vi "Add new Exchange Map.vi"() -> (8 "Long":string, 9 "Lat":string, 10 "Name of University":string, 11 "table id":string)   [LabVIEW 2010]
uses:
  <vilib>/Utility/file.llb/Read From Spreadsheet File (string).vi
panel:
  out "name of logo":string
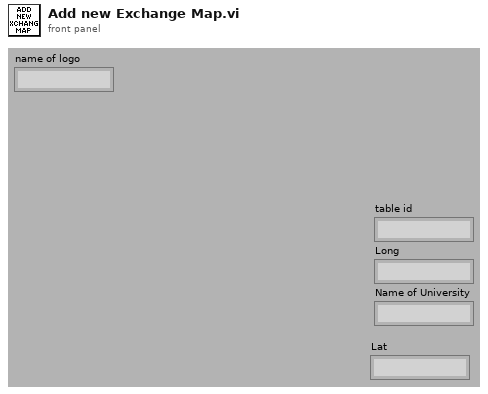
[diagram p1: front panel]
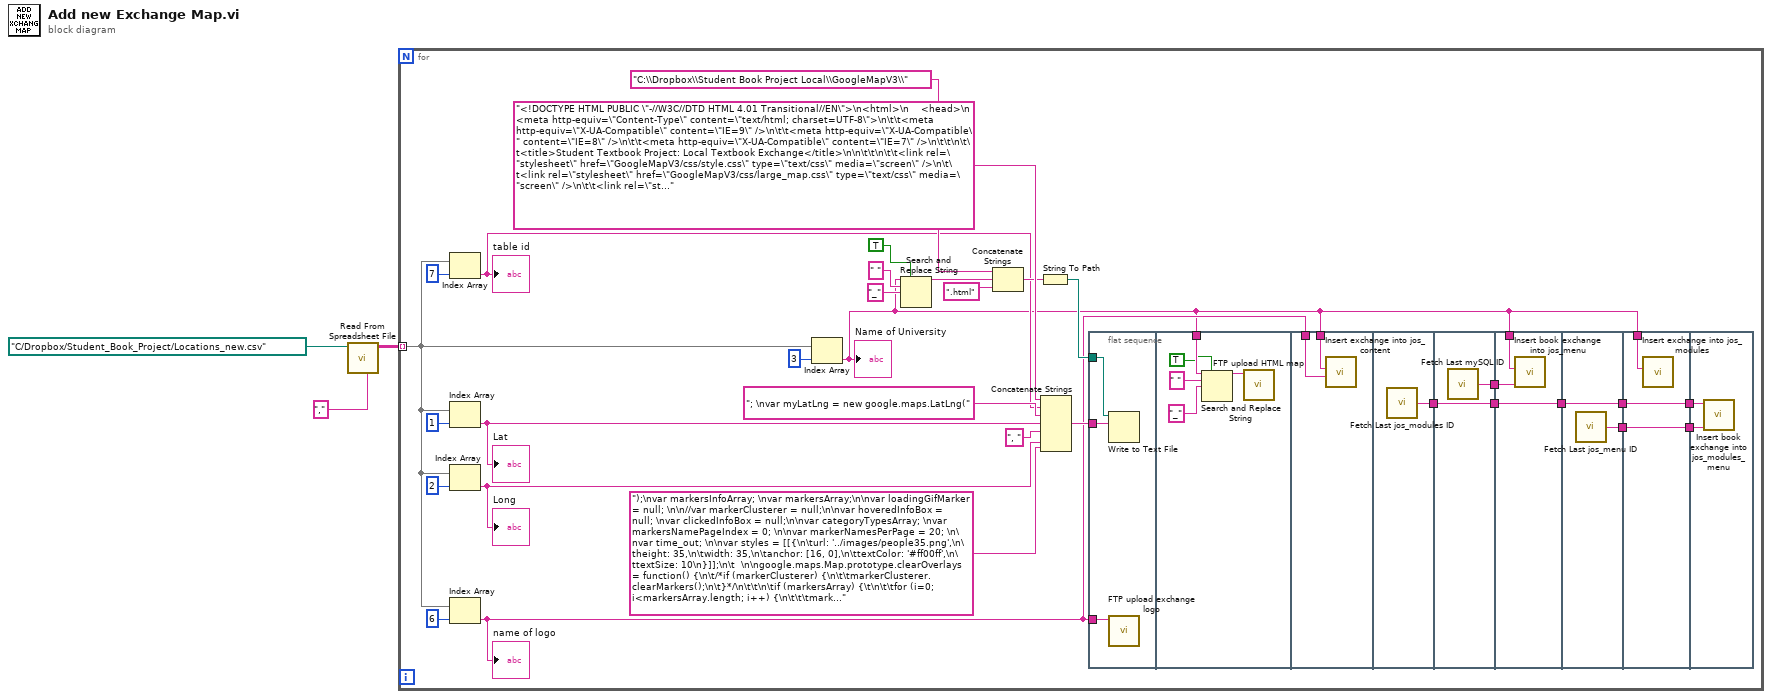
[diagram p0: block diagram]
diagram:
  n1 = call-poly <vilib>:"Read From Spreadsheet File.vi"("delimiter (\\t)"="," ("delimiter (\\t)"), "file path (dialog if empty)"=path "C:/Dropbox/Student_Book_Project/Locations_new.csv") -> ("all rows"=w1:string[][])  [unwired: 5 in, 4 out]
  n2 = for {
    tunnel: w1 -> [w6] mode=indexing
    n3 = Index Array(array=w6, index=7) -> (element=w5:string)
    "table id" <- w5
    n4 = Index Array(array=w6, index=1) -> (element=w13:string)
    "Lat" <- w13
    n5 = Index Array(array=w6, index=2) -> (element=w11:string)
    "Long" <- w11
    n6 = Index Array(array=w6, index=6) -> (element=w7:string)
    "name of logo" <- w7
    n7 = Index Array(array=w6, index=3) -> (element=w4:string)
    "Name of University" <- w4
    n8 = Search and Replace String(replace all?=TRUE ("replace all? (F)"), input string=w4, search string=" ", replace string="_" ("replace string (\"\")")) -> (result string=w15:string)  [unwired: 4 in, 3 out]
    n9 = Concatenate Strings("C:\\Dropbox\\Student Book Project Local\\GoogleMapV3\\", w15, ".html" ("string")) -> (w21:string)
    n10 = String To Path(string=w21) -> (path=w19:path)
    n11 = Concatenate Strings("<!DOCTYPE HTML PUBLIC \"-//W3C//DTD HTML 4.01 Transitional//EN\">\n<html>\n    <head>\n        <meta http-equiv=\"Content-Type\" content=\"text/html; charset=UTF-8\">\n\t\t<meta http-equiv=\"X-UA-Compatible\" content=\"IE=9\" />\n\t\t<meta http-equiv=\"X-UA-Compatible\" content=\"IE=8\" />\n\t\t<meta http-equiv=\"X-UA-Compatible\" content=\"IE=7\" />\n\t\t\n\t\t<title>Student Textbook Project: Local Textbook Exchange</title>\n\n\t\t\n\t\t<link rel=\"stylesheet\" href=\"GoogleMapV3/css/style.css\" type=\"text/css\" media=\"screen\" />\n\t\t<link rel=\"stylesheet\" href=\"GoogleMapV3/css/large_map.css\" type=\"text/css\" media=\"screen\" />\n\t\t<link rel=\"stylesheet\" href=\"GoogleMapV3/css/jquery.customSelect.css\" type=\"text/css\" media=\"screen\" />\n\t\t<link href='http://fonts.googleapis.com/css?family=Happy+Monkey' rel='stylesheet' type='text/css'>\n\t\t<link href='http://fonts.googleapis.com/css?family=Lobster' rel='stylesheet' type='text/css'>\n\t\t<script type=\"text/javascript\" src=\"https://ajax.googleapis.com/ajax/libs/jquery/1.7.1/jquery.min.js\"></script>\n\t\t<!--<script type='text/javascript' src='GoogleMapV3/js/easing.js'></script>-->\n\t\t<script type=\"text/javascript\" src=\"http://maps.google.com/maps/api/js?sensor=false\"></script>\n\t\t<script type=\"text/javascript\" src=\"http://www.google.com/jsapi\"></script>\t\n\n        <script type=\"text/javascript\">\n\t\tvar map;\nvar tableid = ", w5, "; \nvar myLatLng = new google.maps.LatLng(" ("string"), w13, ", " ("string"), w11, ");\nvar markersInfoArray; \nvar markersArray;\n\nvar loadingGifMarker = null; \n\n//var markerClusterer = null;\n\nvar hoveredInfoBox = null; \nvar clickedInfoBox = null;\n\nvar categoryTypesArray; \nvar markersNamePageIndex = 0; \n\nvar markerNamesPerPage = 20; \n\nvar time_out; \n\nvar styles = [[{\n\turl: '../images/people35.png',\n\theight: 35,\n\twidth: 35,\n\tanchor: [16, 0],\n\ttextColor: '#ff00ff',\n\ttextSize: 10\n}]];\n\t  \n\ngoogle.maps.Map.prototype.clearOverlays = function() {\n\t/*if (markerClusterer) {\n\t\tmarkerClusterer.clearMarkers();\n\t}*/\n\t\t\n\tif (markersArray) {\t\n\t\tfor (i=0; i<markersArray.length; i++) {\n\t\t\tmarkersArray[i].setMap(null);\n\t\t}\n\t}\n}\n\ngoogle.load('visualization', '1');\n\n\nfunction initialize()\n{\t\n\t$(\"#controlbtn\").click(function(e) {\n\t\te.preventDefault();\n\t\t\n\t\tvar slidepx=$(\"#srp_left_rail\").width();\n\t\t\n\t\tif ( !$(\"#large_map\").is(':animated') ) { \n\t\t\tif (Math.abs(parseInt($(\"#large_map\").css('marginLeft'), 10)) < slidepx) {\n\t\t\t\t$(this).removeClass('close').html('Hide your stuffs');\n\t\t\t\t\n\t\t\t\tmargin = \"-=\" + slidepx;\n\n\t\t\t} else {\n\t\t\t\t$(this).addClass('close').html('Show your stuffs');\n\t\t\t\t\n\t\t\t\tmargin = \"+=\" + slidepx;\n\n\t\t\t}\n\t\t\n\t\t\t$(\"#large_map\").animate({ \n\t\t\t\tmarginLeft: margin\n\t\t\t}, {\n\t\t\t\t\tduration: 'slow',\n\t\t\t\t\teasing: 'easeOutQuint'\n\t\t\t\t});\t\t\t\t\t\n\t\t} \n\t});\n\t\n\tvar myOptions = {\n\t\tzoom: 14,\n\t\tcenter: myLatLng,\n\t\tmapTypeId: google.maps.MapTypeId.ROADMAP\n\t};\n\tmap = new google.maps.Map(document.getElementById(\"map_canvas\"), myOptions);\n\t\n\tvar query = \"SELECT 'Lat', 'Lng', 'Title', 'Category', 'Price', 'ID' FROM \" + tableid;\n\t\n\tvar queryText = encodeURIComponent(query);\n\tvar gvizQuery = new google.visualization.Query('http://www.google.com/fusiontables/gvizdata?tq=' + queryText);\n\t\n\tmarkersNamePageIndex = 0; \n\tgvizQuery.send(function(response) { \t\n\t\tvar numRows = response.getDataTable().getNumberOfRows();\n\t\t\n\t\t// create the list of lat/long coordinates\n\t\tmarkersInfoArray = [];\n\t\tvar coordinates = [];\n\t\tcategoryTypesArray = [];\n\t\t\n\t\tfor (i=0; i<numRows; i++) {\n\t\t\tvar lat = parseFloat(response.getDataTable().getValue(i, 0));\n\t\t\tvar lng = parseFloat(response.getDataTable().getValue(i, 1));\n\t\t\tvar title = response.getDataTable().getValue(i, 2);\n\t\t\tvar category = response.getDataTable().getValue(i, 3);\n\t\t\tvar price = response.getDataTable().getValue(i, 4);\n\t\t\tvar id = response.getDataTable().getValue(i, 5);\n\t\t\t\n\t\t\tcoordinates.push(new google.maps.LatLng(lat, lng));\n\t\t\n\t\t\tmarkersInfoArray[i] = {id:id, lat:lat, lng:lng, title:title, category:category, price:price};\n\t\t\t\n\t\t\tif (!categoryTypesArray.contains(category)) {\n\t\t\t\tcategoryTypesArray.push(category);\n\t\t\t}\n\t\t}\t\t\t\t\t\n\t\trefreshMarkersCategoryList();\n\t\t\n\t\tmap.clearOverlays();\n\t\tmarkersArray = [];\n\t\t\n\t\tfor (i=0; i<coordinates.length; i++) {\n\t\t\tvar latLng = coordinates[i];\n\t\t\tif (latLng == null) continue; \n\t\t\t\n\t\t\tvar markerInfo = markersInfoArray[i];\n\t\t\tcreateMarker(markerInfo, latLng);\n\t\t}\n\t\t\n\t\t/*var zoom = null; var size = null; var style = null; \n        markerClusterer = new MarkerClusterer(map, markersArray, {\n\t\t\tmaxZoom: zoom,\n\t\t\tgridSize: size,\n\t\t\tstyles: styles[style]\n        });*/\n\t\t\n\t\tvar bounds = new google.maps.LatLngBounds();\n\t\tfor (var i = 0; i < coordinates.length; i++) {\n\t\t\tbounds.extend(coordinates[i]);\n\t\t}\n\t\t\n\t\trefreshMarkersNameList();\n\t});\n}\n\nfunction createMarker(markerInfo, latlng) {\n\tvar id = markerInfo.id;\n\tvar category = markerInfo.category; \n\tvar lat = markerInfo.lat; \n\tvar lng = markerInfo.lng;\n\tvar latLng = new google.maps.LatLng(lat, lng);\n\t\n\tvar color = \"0000FF\"; \n\tif (category == \"History\")\n\t\tcolor = \"0000FF\";\n\telse if (category == \"Film Studies\")\n\t\tcolor = \"FF0000\";\n\telse if (category == \"Biology\")\n\t\tcolor = \"FF9900\"\n\telse if (category == \"Engineering\")\n\t\tcolor = \"E661AC\";\t\t\t\t\t\n\telse if (category == \"Education\")\n\t\tcolor = \"BF94E4\";\n\telse if (category == \"Music\")\n\t\tcolor = \"8E67FD\";\n\telse if (category == \"Chemistry\")\n\t\tcolor = \"804040\";\n\telse if (category == \"Economics\")\n\t\tcolor = \"FF8300\";\n\telse if (category == \"Political Science\")\n\t\tcolor = \"000000\";\n\telse if (category == \"Medical\")\n\t\tcolor = \"00FF00\";\n\telse if (category == \"Mathematics\")\n\t\tcolor = \"06DCFB\";\t\n\telse if (category == \"Psychology\")\n\t\tcolor = \"FF68DD\"; \n\telse if (category == \"Uncategorized\")\n\t\tcolor = \"1FCB4A\";\n\telse if (category == \"Physics\")\n\t\tcolor = \"800080\"; \n\telse if (category == \"Language\")\n\t\tcolor = \"804040\"; \n\telse if (category == \"Hospitality Management\")\n\t\tcolor = \"988727\"; \n\telse if (category == \"Nursing\")\n\t\tcolor = \"808080\"; \n\telse if (category == \"Business\")\n\t\tcolor = \"0080FF\"; \n\telse if (category == \"Art\")\n\t\tcolor = \"FF8080\"; \n\t\n\tvar markerString = markerInfo.price.toString();\n\t\n\tvar marker = new google.maps.Marker({\n\t\tposition: latlng,\n\t\tdraggable: false,\n\t\tmap: map,\n\t\ticon: new google.maps.MarkerImage(\"http://chart.googleapis.com/chart?chst=d_bubble_text_small&chld=bb|\"+markerString+\"|\"+color+\"|FFFFFF\", null, null, new google.maps.Point(15, 42)),\n\t\tshadow: new google.maps.MarkerImage(\"http://chart.googleapis.com/chart?chst=d_bubble_text_small_shadow&chld=bb|\"+markerString, null, null, new google.maps.Point(15, 45))\n\t});\n\tmarker.set(\"id\", id);\n\t\n\tmarkersArray.push(marker);\t\t\t\t\n\t\n\t// when hovering the bookstore ...\t\n\tgoogle.maps.event.addListener(marker, \"mouseover\", function(e) {\n\t\tvar id = marker.get(\"id\");\n\t\tvar query = \"SELECT 'Date', 'Time', 'Lat', 'Lng', 'Title', 'Category', 'Author', 'ISBN', 'Price', 'Class Identifier', 'Condition', 'Contact Info', 'Meta', 'Extra Information', 'Username', 'UserID', 'Name', 'Address', 'City', 'State', 'Zip Code', 'Country', 'timestamp', 'ID' FROM \" + tableid + \" WHERE ID='\" + id + \"'\";\n\t\t\n\t\tvar queryText = encodeURIComponent(query);\n\t\tvar gvizQuery = new google.visualization.Query('http://www.google.com/fusiontables/gvizdata?tq=' + queryText);\n\t\t\n\t\tgvizQuery.send(function(response) { \t\n\t\t\tvar numRows = response.getDataTable().getNumberOfRows();\n\t\t\t\n\t\t\tfor (i=0; i<numRows; i++) {\n\t\t\t\tvar date = response.getDataTable().getValue(i, 0);\n\t\t\t\tvar time = response.getDataTable().getValue(i, 1);\n\t\t\t\tvar lat = parseFloat(response.getDataTable().getValue(i, 2));\n\t\t\t\tvar lng = parseFloat(response.getDataTable().getValue(i, 3));\n\t\t\t\tvar title = response.getDataTable().getValue(i, 4);\n\t\t\t\tvar category = response.getDataTable().getValue(i, 5);\n\t\t\t\tvar author = response.getDataTable().getValue(i, 6);\n\t\t\t\tvar isbn = response.getDataTable().getValue(i, 7);\n\t\t\t\tvar price = response.getDataTable().getValue(i, 8);\n\t\t\t\tvar class_identifier = response.getDataTable().getValue(i, 9);\n\t\t\t\tvar condition = response.getDataTable().getValue(i, 10);\n\t\t\t\tvar contact_info = response.getDataTable().getValue(i, 11);\n\t\t\t\tvar meta = response.getDataTable().getValue(i, 12);\n\t\t\t\tvar extra_information = response.getDataTable().getValue(i, 13);\n\t\t\t\tvar username = response.getDataTable().getValue(i, 14);\n\t\t\t\tvar userid = response.getDataTable().getValue(i, 15);\n\t\t\t\tvar name = response.getDataTable().getValue(i, 16);\n\t\t\t\tvar address = response.getDataTable().getValue(i, 17);\n\t\t\t\tvar city = response.getDataTable().getValue(i, 18);\n\t\t\t\tvar state = response.getDataTable().getValue(i, 19);\n\t\t\t\tvar zipcode = response.getDataTable().getValue(i, 20);\n\t\t\t\tvar country = response.getDataTable().getValue(i, 21);\n\t\t\t\tvar timestamp = response.getDataTable().getValue(i, 22);\n\t\t\t\tvar id = response.getDataTable().getValue(i, 23);\n\t\t\t\t\n\t\t\t\tvar hoveredBoxText = document.createElement(\"div\");\n\t\t\t\thoveredBoxText.style.cssText = \"border: 1px solid black; margin-top: 8px; background:#333; color:#FFF; font-family: 'Happy Monkey', cursive; font-size:12px; padding: 5px; border-radius:8px; -moz-border-radius:8px; -webkit-border-radius:8px; behavior: url(ie-css3.htc);\";\n\t\t\t\thoveredBoxText.innerHTML = '<div style=\"height:400px; overflow:auto;\"><p style=\"font-size:16px; font-weight:bold; color:#3990BD; margin-top:0px; margin-bottom:-10px;\">' + title + '</p>' + \n\t\t\t\t\t\t\t\"<br /><br /><strong>Category</strong>:  \" + category + \n\t\t\t\t\t\t\t\"<br /><strong>Author</strong>:  \" + author + \n\t\t\t\t\t\t\t\"<br /><strong>ISBN</strong>:  \" + isbn + \n\t\t\t\t\t\t\t\"<br /><strong>Price</strong>:  \" + price + \n\t\t\t\t\t\t\t\"<br /><strong>Class Identifier</strong>:  \" + class_identifier + \n\t\t\t\t\t\t\t\"<br /><strong>Condition</strong>:  \" + condition + \n\t\t\t\t\t\t\t\"<br /><strong>Contact Info</strong>:  \" + contact_info + \n\t\t\t\t\t\t\t\"<br />  \" + extra_information + '</div>';\n\t\t\t\t\n\t\t\t\tvar hoveredInfoBoxOptions = {\n\t\t\t\t\tcontent: hoveredBoxText\n\t\t\t\t\t,disableAutoPan: false\n\t\t\t\t\t,maxWidth: 0\n\t\t\t\t\t,pixelOffset: new google.maps.Size(-133, 0)\n\t\t\t\t\t,zIndex: 100000\n\t\t\t\t\t,boxStyle: { \n\t\t\t\t\t\tbackground: \"url('GoogleMapV3/images/tipbox.gif') no-repeat\"\n\t\t\t\t\t\t,opacity: 0.94\n\t\t\t\t\t\t,width: \"350px\"\n\t\t\t\t\t\t,height: \"400px\"\t\t\t\t\t\t\t\n\t\t\t\t\t}\n\t\t\t\t\t,closeBoxMargin: \"15px 7px 7px 7px\"\n\t\t\t\t\t,closeBoxURL: \"http://www.google.com/intl/en_us/mapfiles/close.gif\"\n\t\t\t\t\t,infoBoxClearance: new google.maps.Size(1, 1)\n\t\t\t\t\t,isHidden: false\n\t\t\t\t\t,pane: \"floatPane\"\n\t\t\t\t\t,enableEventPropagation: false\n\t\t\t\t\t,disableAutoPan: true\n\t\t\t\t};\n\t\t\t\t\n\t\t\t\tif (hoveredInfoBox != null)\n\t\t\t\t\thoveredInfoBox.close(); \n\t\t\t\t\t\t\n\t\t\t\tif (hoveredInfoBox == null)\n\t\t\t\t\thoveredInfoBox = new InfoBox(hoveredInfoBoxOptions);\n\t\t\t\telse {\n\t\t\t\t\thoveredInfoBox.setContent(hoveredBoxText);\t\t\t\t\t\t\n\t\t\t\t\thoveredInfoBox.setZIndex(100000);\n\t\t\t\t}\n\t\t\t\t\t\n\t\t\t\thoveredInfoBox.setContent(hoveredBoxText);\t\t\t\t\t\t\n\t\t\t\thoveredInfoBox.setZIndex(100000);\n\t\t\t\thoveredInfoBox.open(map, marker);\n\t\t\t}\n\t\t});\n\t});\n\t\n\tgoogle.maps.event.addListener(marker, \"mouseout\", function(e) {\t\t\n\t\thoveredInfoBox.close();\n\t});\n\t\n\t// when clicking the bookstore ...\t\n\tgoogle.maps.event.addListener(marker, \"click\", function(e) {\n\t\tvar id = marker.get(\"id\");\n\t\tvar query = \"SELECT 'Date', 'Time', 'Lat', 'Lng', 'Title', 'Category', 'Author', 'ISBN', 'Price', 'Class Identifier', 'Condition', 'Contact Info', 'Meta', 'Extra Information', 'Username', 'UserID', 'Name', 'Address', 'City', 'State', 'Zip Code', 'Country', 'timestamp', 'ID' FROM \" + tableid + \" WHERE ID='\" + id + \"'\";\n\t\t\n\t\tvar queryText = encodeURIComponent(query);\n\t\tvar gvizQuery = new google.visualization.Query('http://www.google.com/fusiontables/gvizdata?tq=' + queryText);\n\t\t\n\t\tgvizQuery.send(function(response) { \t\n\t\t\tvar numRows = response.getDataTable().getNumberOfRows();\n\t\t\t\n\t\t\tfor (i=0; i<numRows; i++) {\n\t\t\t\tvar date = response.getDataTable().getValue(i, 0);\n\t\t\t\tvar time = response.getDataTable().getValue(i, 1);\n\t\t\t\tvar lat = parseFloat(response.getDataTable().getValue(i, 2));\n\t\t\t\tvar lng = parseFloat(response.getDataTable().getValue(i, 3));\n\t\t\t\tvar title = response.getDataTable().getValue(i, 4);\n\t\t\t\tvar category = response.getDataTable().getValue(i, 5);\n\t\t\t\tvar author = response.getDataTable().getValue(i, 6);\n\t\t\t\tvar isbn = response.getDataTable().getValue(i, 7);\n\t\t\t\tvar price = response.getDataTable().getValue(i, 8);\n\t\t\t\tvar class_identifier = response.getDataTable().getValue(i, 9);\n\t\t\t\tvar condition = response.getDataTable().getValue(i, 10);\n\t\t\t\tvar contact_info = response.getDataTable().getValue(i, 11);\n\t\t\t\tvar meta = response.getDataTable().getValue(i, 12);\n\t\t\t\tvar extra_information = response.getDataTable().getValue(i, 13);\n\t\t\t\tvar username = response.getDataTable().getValue(i, 14);\n\t\t\t\tvar userid = response.getDataTable().getValue(i, 15);\n\t\t\t\tvar name = response.getDataTable().getValue(i, 16);\n\t\t\t\tvar address = response.getDataTable().getValue(i, 17);\n\t\t\t\tvar city = response.getDataTable().getValue(i, 18);\n\t\t\t\tvar state = response.getDataTable().getValue(i, 19);\n\t\t\t\tvar zipcode = response.getDataTable().getValue(i, 20);\n\t\t\t\tvar country = response.getDataTable().getValue(i, 21);\n\t\t\t\tvar timestamp = response.getDataTable().getValue(i, 22);\n\t\t\t\tvar id = response.getDataTable().getValue(i, 23);\n\t\t\t\t\n\t\t\t\t// clicked info bubble ...\n\t\t\t\tvar clickedBoxText = document.createElement(\"div\");\n\t\t\t\tclickedBoxText.style.cssText = \"border: 1px solid black; margin-top: 8px; background:#333; color:#FFF; font-family: 'Happy Monkey', cursive; font-size:12px; padding: 5px; border-radius:8px; -webkit-border-radius:8px; -moz-border-radius:8px;\";\n\t\t\t\tclickedBoxText.innerHTML = '<div style=\"height:400px; overflow:auto;\"><p style=\"font-size:16px; font-weight:bold; color:#3990BD; margin-top:0px; margin-bottom:-10px;\">' + title + '</p>' + \n\t\t\t\t\t\t\t\"<br /><br /><strong>Category</strong>:  \" + category + \n\t\t\t\t\t\t\t\"<br /><strong>Author</strong>:  \" + author + \n\t\t\t\t\t\t\t\"<br /><strong>ISBN</strong>:  \" + isbn + \n\t\t\t\t\t\t\t\"<br /><strong>Price</strong>:  \" + price + \n\t\t\t\t\t\t\t\"<br /><strong>Class Identifier</strong>:  \" + class_identifier + \n\t\t\t\t\t\t\t\"<br /><strong>Condition</strong>:  \" + condition + \n\t\t\t\t\t\t\t\"<br /><strong>Contact Info</strong>:  \" + contact_info + \n\t\t\t\t\t\t\t\"<br />  \" + extra_information + '</div>';\n\t\t\t\t\n\t\t\t\tvar clickedInfoBoxOptions = {\n\t\t\t\t\tcontent: clickedBoxText\n\t\t\t\t\t,disableAutoPan: false\n\t\t\t\t\t,maxWidth: 0\n\t\t\t\t\t,pixelOffset: new google.maps.Size(-133, 0)\n\t\t\t\t\t,zIndex: 100000\n\t\t\t\t\t,boxStyle: { \n\t\t\t\t\t\tbackground: \"url('GoogleMapV3/images/tipbox.gif') no-repeat\"\n\t\t\t\t\t\t,opacity: 0.94\n\t\t\t\t\t\t,width: \"400px\"\n\t\t\t\t\t\t,height: \"450px\"\t\t\t\t\t\t\t\n\t\t\t\t\t}\n\t\t\t\t\t,closeBoxMargin: \"15px 7px 7px 7px\"\n\t\t\t\t\t,closeBoxURL: \"http://www.google.com/intl/en_us/mapfiles/close.gif\"\n\t\t\t\t\t,infoBoxClearance: new google.maps.Size(1, 1)\n\t\t\t\t\t,isHidden: false\n\t\t\t\t\t,pane: \"floatPane\"\n\t\t\t\t\t,enableEventPropagation: false\n\t\t\t\t};\n\t\t\t\t\n\t\t\t\tif (clickedInfoBox == null)\n\t\t\t\t\tclickedInfoBox = new InfoBox(clickedInfoBoxOptions);\n\t\t\t\telse {\n\t\t\t\t\tclickedInfoBox.setContent(clickedBoxText);\t\t\t\t\t\t\n\t\t\t\t\tclickedInfoBox.setZIndex(100000);\n\t\t\t\t}\n\t\t\t\t\n\t\t\t\tif (hoveredInfoBox != null)\n\t\t\t\t\thoveredInfoBox.close(); \n\t\t\t\tif (clickedInfoBox != null)\n\t\t\t\t\tclickedInfoBox.close();\n\t\t\t\t\t\n\t\t\t\tclickedInfoBox.setContent(clickedBoxText);\t\t\t\t\t\t\n\t\t\t\tclickedInfoBox.setZIndex(100000);\n\t\t\t\t\n\t\t\t\tclickedInfoBox.open(map, marker);\n\t\t\t}\n\t\t});\n\t});\n}\n\nfunction refreshMarkersCategoryList() { \n\tcategoryTypesArray.sort(sortNumber);\n\t\n\tvar marker_categories_select = document.getElementById('marker_categories');\n\taddSelectOption(marker_categories_select, \"All\", 0, true);\n\t\n\tfor (i=0; i<categoryTypesArray.length; i++) {\n\t\tvar added_current_category = categoryTypesArray[i];\n\t\taddSelectOption(marker_categories_select, added_current_category, added_current_category, false);\n\t}\n} \n\nfunction refreshMarkersNameList() { \n\t\n\tvar marker_titles_add_html = \"\";\t\t\t\t\n\t\n\tvar markersNum = markersInfoArray.length; \n\tvar markerInfo; var markerName; var markerId; \n\tif (markersNum > markerNamesPerPage) {\n\t\tfor (i=0; i<markerNamesPerPage; i++) {\n\t\t\tif ( (i + markersNamePageIndex * markerNamesPerPage) >= markersNum )\n\t\t\t\tbreak;\n\t\t\t\t\n\t\t\tmarkerInfo = markersInfoArray[i + markersNamePageIndex * markerNamesPerPage];\n\t\t\tmarkerTitle = markerInfo.title; \n\t\t\tmarkerId = markerInfo.id;\n\t\t\t\n\t\t\tmarker_titles_add_html += '<li><a title=\"' + markerTitle + '\" href=\"javascript:void(0);\" onmouseover=\"openMarkerNameInfoWindowOnMap(' + markerId + ')\" onmouseout=\"closeMarkerNameInfoWindowOnMap(' + markerId + ')\" onclick=\"selectMarkerInfoOnMap(' + markerId + ')\">' + markerTitle + '</a></li>'\n\t\t}\n\t\t\n\t\tvar marker_names_prev_next_html = \"\";\n\t\tmarker_names_prev_next_html += '<a href=\"javascript:void(0);\" onclick=\"showPrevMarkerNames();\" style=\"margin-left:40px;\"><< Previous</a>'\n\t\tmarker_names_prev_next_html += '<a href=\"javascript:void(0);\" onclick=\"showNextMarkerNames();\" style=\"margin-left:60px;\">Next >></a>'\n\n\t\tdocument.getElementById('markers_prev_next_section').innerHTML = marker_names_prev_next_html; \n\t} else {\n\t\tfor (i=0; i<markersNum; i++) {\n\t\t\tmarkerInfo = markersInfoArray[i];\n\t\t\tmarkerTitle = markerInfo.title; \n\t\t\tmarkerId = markerInfo.id;\n\t\t\t\n\t\t\tmarker_titles_add_html += '<li><a title=\"' + markerName + '\" href=\"javascript:void(0);\" onmouseover=\"openMarkerNameInfoWindowOnMap(' + markerId + ')\" onmouseout=\"closeMarkerNameInfoWindowOnMap(' + markerId + ')\" onclick=\"selectMarkerInfoOnMap(' + markerId + ')\">' + markerTitle + '</a></li>'\n\t\t}\n\t\t\n\t\tdocument.getElementById('markers_prev_next_section').innerHTML = \"\"; \n\t}\n\tdocument.getElementById('markers_list').innerHTML = marker_titles_add_html; \n}\n\nfunction showPrevMarkerNames() { \n\tif (markersNamePageIndex == 0)\n\t\treturn;\n\t\t\n\tmarkersNamePageIndex--;\n\trefreshMarkersNameList();\n}\n\nfunction showNextMarkerNames() { \n\tvar markersNum = markersInfoArray.length; \n\tif ( ((markersNamePageIndex+1) * markerNamesPerPage) > markersNum ) \n\t\treturn; \n\t\t\n\tmarkersNamePageIndex++;\n\trefreshMarkersNameList();\n}\n\nfunction SearchBooks(search_text, search_category) {\n\tsearch_text = trim(search_text.toString());\n\t\n\tvar query = \"\"; \n\t\n\tif (search_category == 0)\n\t\tquery = \"SELECT 'Lat', 'Lng', 'Title', 'Category', 'Price', 'ID' FROM \" + tableid;\n\telse \n\t\tquery = \"SELECT 'Lat', 'Lng', 'Title', 'Category', 'Price', 'ID' FROM \" + tableid + \" WHERE Category='\" + search_category.toString() + \"'\";\n\t\t\n\tvar queryText = encodeURIComponent(query);\n\tvar gvizQuery = new google.visualization.Query('http://www.google.com/fusiontables/gvizdata?tq='  + queryText);\n\t\n\tmarkersNamePageIndex = 0; \n\t\n\t// Send query and draw table with data in response\n\tgvizQuery.send(function(response) {\n\t\tvar numRows = response.getDataTable().getNumberOfRows();\n\t\tvar numCols = response.getDataTable().getNumberOfColumns();\n\t\t\n\t\t// create the list of lat/long coordinates\n\t\tmarkersInfoArray = [];\n\t\tvar coordinates = [];\n\t\t\n\t\tvar is_match = false; \n\t\t\n\t\tvar index = 0; \n\t\tfor (i=0; i<numRows; i++) {\n\t\t\tis_match = false;\n\n\t\t\tvar lat = parseFloat(response.getDataTable().getValue(i, 0));\n\t\t\tvar lng = parseFloat(response.getDataTable().getValue(i, 1));\n\t\t\tvar title = response.getDataTable().getValue(i, 2);\n\t\t\tvar category = response.getDataTable().getValue(i, 3);\n\t\t\tvar price = response.getDataTable().getValue(i, 4);\n\t\t\tvar id = response.getDataTable().getValue(i, 5);\n\t\t\t\n\t\t\tif (search_text != \"\") {\n\t\t\t\tis_match = isMatchWithSearchText(search_text, title, category, price, id);\n\t\t\t\tif (is_match == false)\n\t\t\t\t\tcontinue; \n\t\t\t\t\n\t\t\t\tcoordinates.push(new google.maps.LatLng(lat, lng));\n\t\t\t\t\n\t\t\t\tmarkersInfoArray[index] = {id:id, lat:lat, lng:lng, title:title, category:category, price:price};\n\t\t\t\t\n\t\t\t\tindex++;\n\t\t\t\t\n\t\t\t\tcontinue; \n\t\t\t}\n\t\t\t\n\t\t\tcoordinates.push(new google.maps.LatLng(lat, lng));\n\t\t\tmarkersInfoArray[i] = {id:id, lat:lat, lng:lng, title:title, category:category, price:price};\n\t\t}\t\t\n\t\t\n\t\tmap.clearOverlays();\n\t\tmarkersArray = [];\n\t\t\n\t\tfor (i=0; i<coordinates.length; i++) {\n\t\t\tvar latLng = coordinates[i];\n\t\t\tif (latLng == null) continue; \n\t\t\t\n\t\t\tvar markerInfo = markersInfoArray[i];\n\t\t\n\t\t\tcreateMarker(markerInfo, latLng);\n\t\t}\n\t\t\n\t\t/*var zoom = null; var size = null; var style = null; \t\t\n\t\tmarkerClusterer = new MarkerClusterer(map, markersArray, {\n\t\t\tmaxZoom: zoom,\n\t\t\tgridSize: size,\n\t\t\tstyles: styles[style]\n        });*/\n\t\t\n\t\tvar bounds = new google.maps.LatLngBounds();\n\t\tfor (var i = 0; i < coordinates.length; i++) {\n\t\t\tbounds.extend(coordinates[i]);\n\t\t}\n\t\tmap.fitBounds(bounds);\n\t\t\n\t\trefreshMarkersNameList();\n\t});\n}\n\nfunction isMatchWithSearchText(search_text, title, category, price, id) {\n\t\n\tsearch_text = search_text.toLowerCase();\n\t\n\tvar strTitle = trim(String(title));\n\tstrTitle = strTitle.toLowerCase();\n\t\n\tvar strCategory = trim(String(category));\n\tstrCategory = strCategory.toLowerCase();\n\t\n\tif (strTitle.indexOf(search_text) !== -1)\n\t\treturn true;\n\t\t\n\treturn false; \n}\n\nfunction openMarkerNameInfoWindowOnMap(markerId) {\n\tvar query = \"SELECT 'Date', 'Time', 'Lat', 'Lng', 'Title', 'Category', 'Author', 'ISBN', 'Price', 'Class Identifier', 'Condition', 'Contact Info', 'Meta', 'Extra Information', 'Username', 'UserID', 'Name', 'Address', 'City', 'State', 'Zip Code', 'Country', 'timestamp', 'ID' FROM \" + tableid + \" WHERE ID='\" + markerId + \"'\";\n\t\t\n\tvar queryText = encodeURIComponent(query);\n\tvar gvizQuery = new google.visualization.Query('http://www.google.com/fusiontables/gvizdata?tq=' + queryText);\n\t\n\tgvizQuery.send(function(response) { \t\n\t\tvar numRows = response.getDataTable().getNumberOfRows();\n\t\tfor (var i=0; i<numRows; i++) {\n\t\t\tvar date = response.getDataTable().getValue(i, 0);\n\t\t\tvar time = response.getDataTable().getValue(i, 1);\n\t\t\tvar lat = parseFloat(response.getDataTable().getValue(i, 2));\n\t\t\tvar lng = parseFloat(response.getDataTable().getValue(i, 3));\n\t\t\tvar title = response.getDataTable().getValue(i, 4);\n\t\t\tvar category = response.getDataTable().getValue(i, 5);\n\t\t\tvar author = response.getDataTable().getValue(i, 6);\n\t\t\tvar isbn = response.getDataTable().getValue(i, 7);\n\t\t\tvar price = response.getDataTable().getValue(i, 8);\n\t\t\tvar class_identifier = response.getDataTable().getValue(i, 9);\n\t\t\tvar condition = response.getDataTable().getValue(i, 10);\n\t\t\tvar contact_info = response.getDataTable().getValue(i, 11);\n\t\t\tvar meta = response.getDataTable().getValue(i, 12);\n\t\t\tvar extra_information = response.getDataTable().getValue(i, 13);\n\t\t\tvar username = response.getDataTable().getValue(i, 14);\n\t\t\tvar userid = response.getDataTable().getValue(i, 15);\n\t\t\tvar name = response.getDataTable().getValue(i, 16);\n\t\t\tvar address = response.getDataTable().getValue(i, 17);\n\t\t\tvar city = response.getDataTable().getValue(i, 18);\n\t\t\tvar state = response.getDataTable().getValue(i, 19);\n\t\t\tvar zipcode = response.getDataTable().getValue(i, 20);\n\t\t\tvar country = response.getDataTable().getValue(i, 21);\n\t\t\tvar timestamp = response.getDataTable().getValue(i, 22);\n\t\t\tvar id = response.getDataTable().getValue(i, 23);\n\t\t\t\n\t\t\t\n\t\t\tvar marker = null; \n\t\t\tvar markerId = -1; \n\t\t\tfor (var j=0; j<markersArray.length; j++)\n\t\t\t{\n\t\t\t\tmarker = markersArray[j]; \n\t\t\t\tmarkerId = marker.get(\"id\");\n\t\t\t\tif (markerId == id)\n\t\t\t\t\tbreak;\n\t\t\t}\n\t\t\tif (marker == null)\n\t\t\t\treturn;\n\t\t\t\n\t\t\tvar hoveredBoxText = document.createElement(\"div\");\n\t\t\thoveredBoxText.style.cssText = \"border: 1px solid black; margin-top: 8px; background:#333; color:#FFF; font-family: 'Happy Monkey', cursive; font-size:12px; padding: 5px; border-radius:8px; -moz-border-radius:8px; -webkit-border-radius:8px; behavior: url(ie-css3.htc);\";\n\t\t\thoveredBoxText.innerHTML = '<div style=\"height:400px; overflow:auto;\"><p style=\"font-size:16px; font-weight:bold; color:#3990BD; margin-top:0px; margin-bottom:-10px;\">' + title + '</p>' + \n\t\t\t\t\t\t\"<br /><br /><strong>Category</strong>:  \" + category + \n\t\t\t\t\t\t\"<br /><strong>Author</strong>:  \" + author + \n\t\t\t\t\t\t\"<br /><strong>ISBN</strong>:  \" + isbn + \n\t\t\t\t\t\t\"<br /><strong>Price</strong>:  \" + price + \n\t\t\t\t\t\t\"<br /><strong>Class Identifier</strong>:  \" + class_identifier + \n\t\t\t\t\t\t\"<br /><strong>Condition</strong>:  \" + condition + \n\t\t\t\t\t\t\"<br /><strong>Contact Info</strong>:  \" + contact_info + \n\t\t\t\t\t\t\"<br />  \" + extra_information + '</div>';\n\t\t\t\n\t\t\tvar hoveredInfoBoxOptions = {\n\t\t\t\tcontent: hoveredBoxText\n\t\t\t\t,disableAutoPan: false\n\t\t\t\t,maxWidth: 0\n\t\t\t\t,pixelOffset: new google.maps.Size(-133, 0)\n\t\t\t\t,zIndex: 100000\n\t\t\t\t,boxStyle: { \n\t\t\t\t\tbackground: \"url('GoogleMapV3/images/tipbox.gif') no-repeat\"\n\t\t\t\t\t,opacity: 0.94\n\t\t\t\t\t,width: \"400px\"\n\t\t\t\t\t,height: \"450px\"\t\t\t\t\t\t\t\n\t\t\t\t}\n\t\t\t\t,closeBoxMargin: \"15px 7px 7px 7px\"\n\t\t\t\t,closeBoxURL: \"http://www.google.com/intl/en_us/mapfiles/close.gif\"\n\t\t\t\t,infoBoxClearance: new google.maps.Size(1, 1)\n\t\t\t\t,isHidden: false\n\t\t\t\t,pane: \"floatPane\"\n\t\t\t\t,enableEventPropagation: false\n\t\t\t\t,disableAutoPan: true\n\t\t\t};\n\t\t\n\t\t\tif (hoveredInfoBox != null)\n\t\t\t\thoveredInfoBox.close(); \n\t\t\t\t\t\n\t\t\tif (hoveredInfoBox == null)\n\t\t\t\thoveredInfoBox = new InfoBox(hoveredInfoBoxOptions);\n\t\t\telse {\n\t\t\t\thoveredInfoBox.setContent(hoveredBoxText);\t\t\t\t\t\t\n\t\t\t\thoveredInfoBox.setZIndex(100000);\n\t\t\t}\n\t\t\t\n\t\t\thoveredInfoBox.setContent(hoveredBoxText);\t\t\t\t\t\t\n\t\t\thoveredInfoBox.setZIndex(100000);\n\t\t\thoveredInfoBox.open(map, marker);\n\t\t}\n\t});\n}\n\nfunction closeMarkerNameInfoWindowOnMap(markerId) {\n\thoveredInfoBox.close();\n}\n\nfunction selectMarkerInfoOnMap(markerId) {\n\tvar query = \"SELECT 'Date', 'Time', 'Lat', 'Lng', 'Title', 'Category', 'Author', 'ISBN', 'Price', 'Class Identifier', 'Condition', 'Contact Info', 'Meta', 'Extra Information', 'Username', 'UserID', 'Name', 'Address', 'City', 'State', 'Zip Code', 'Country', 'timestamp', 'ID' FROM \" + tableid + \" WHERE ID='\" + markerId + \"'\";\n\t\t\n\tvar queryText = encodeURIComponent(query);\n\tvar gvizQuery = new google.visualization.Query('http://www.google.com/fusiontables/gvizdata?tq=' + queryText);\n\t\n\tgvizQuery.send(function(response) { \t\n\t\tvar numRows = response.getDataTable().getNumberOfRows();\n\t\t\n\t\tfor (i=0; i<numRows; i++) {\n\t\t\tvar date = response.getDataTable().getValue(i, 0);\n\t\t\tvar time = response.getDataTable().getValue(i, 1);\n\t\t\tvar lat = parseFloat(response.getDataTable().getValue(i, 2));\n\t\t\tvar lng = parseFloat(response.getDataTable().getValue(i, 3));\n\t\t\tvar title = response.getDataTable().getValue(i, 4);\n\t\t\tvar category = response.getDataTable().getValue(i, 5);\n\t\t\tvar author = response.getDataTable().getValue(i, 6);\n\t\t\tvar isbn = response.getDataTable().getValue(i, 7);\n\t\t\tvar price = response.getDataTable().getValue(i, 8);\n\t\t\tvar class_identifier = response.getDataTable().getValue(i, 9);\n\t\t\tvar condition = response.getDataTable().getValue(i, 10);\n\t\t\tvar contact_info = response.getDataTable().getValue(i, 11);\n\t\t\tvar meta = response.getDataTable().getValue(i, 12);\n\t\t\tvar extra_information = response.getDataTable().getValue(i, 13);\n\t\t\tvar username = response.getDataTable().getValue(i, 14);\n\t\t\tvar userid = response.getDataTable().getValue(i, 15);\n\t\t\tvar name = response.getDataTable().getValue(i, 16);\n\t\t\tvar address = response.getDataTable().getValue(i, 17);\n\t\t\tvar city = response.getDataTable().getValue(i, 18);\n\t\t\tvar state = response.getDataTable().getValue(i, 19);\n\t\t\tvar zipcode = response.getDataTable().getValue(i, 20);\n\t\t\tvar country = response.getDataTable().getValue(i, 21);\n\t\t\tvar timestamp = response.getDataTable().getValue(i, 22);\n\t\t\tvar id = response.getDataTable().getValue(i, 23);\n\t\t\t\n\t\t\tvar marker = null; \n\t\t\tvar markerId = -1; \n\t\t\tfor (var j=0; j<markersArray.length; j++)\n\t\t\t{\n\t\t\t\tmarker = markersArray[j]; \n\t\t\t\tmarkerId = marker.get(\"id\");\n\t\t\t\tif (markerId == id)\n\t\t\t\t\tbreak;\n\t\t\t}\n\t\t\tif (marker == null)\n\t\t\t\treturn;\n\t\t\t\t\n\t\t\tvar clickedBoxText = document.createElement(\"div\");\n\t\t\tclickedBoxText.style.cssText = \"border: 1px solid black; margin-top: 8px; background:#333; color:#FFF; font-family: 'Happy Monkey', cursive; font-size:12px; padding: 5px; border-radius:8px; -webkit-border-radius:8px; -moz-border-radius:8px;\";\n\t\t\tclickedBoxText.innerHTML = '<div style=\"height:400px; overflow:auto;\"><p style=\"font-size:16px; font-weight:bold; color:#3990BD; margin-top:0px; margin-bottom:-10px;\">' + title + '</p>' + \n\t\t\t\t\t\"<br /><br /><strong>Category</strong>:  \" + category + \n\t\t\t\t\t\"<br /><strong>Author</strong>:  \" + author + \n\t\t\t\t\t\"<br /><strong>ISBN</strong>:  \" + isbn + \n\t\t\t\t\t\"<br /><strong>Price</strong>:  \" + price + \n\t\t\t\t\t\"<br /><strong>Class Identifier</strong>:  \" + class_identifier + \n\t\t\t\t\t\"<br /><strong>Condition</strong>:  \" + condition + \n\t\t\t\t\t\"<br /><strong>Contact Info</strong>:  \" + contact_info + \n\t\t\t\t\t\"<br />  \" + extra_information + '</div>';\n\t\t\t\n\t\t\tvar clickedInfoBoxOptions = {\n\t\t\t\tcontent: clickedBoxText\n\t\t\t\t,disableAutoPan: false\n\t\t\t\t,maxWidth: 0\n\t\t\t\t,pixelOffset: new google.maps.Size(-133, 0)\n\t\t\t\t,zIndex: 1000\n\t\t\t\t,boxStyle: { \n\t\t\t\t\tbackground: \"url('GoogleMapV3/images/tipbox.gif') no-repeat\"\n\t\t\t\t\t,opacity: 0.94\n\t\t\t\t\t,width: \"400px\"\n\t\t\t\t\t,height: \"450px\"\t\t\t\t\t\t\t\n\t\t\t\t}\n\t\t\t\t,closeBoxMargin: \"15px 7px 7px 7px\"\n\t\t\t\t,closeBoxURL: \"http://www.google.com/intl/en_us/mapfiles/close.gif\"\n\t\t\t\t,infoBoxClearance: new google.maps.Size(1, 1)\n\t\t\t\t,isHidden: false\n\t\t\t\t,pane: \"floatPane\"\n\t\t\t\t,enableEventPropagation: false\n\t\t\t};\n\t\t\t\n\t\t\tif (hoveredInfoBox != null)\n\t\t\t\thoveredInfoBox.close(); \n\t\t\tif (clickedInfoBox != null)\n\t\t\t\tclickedInfoBox.close();\n\t\t\t\t\t\n\t\t\tif (clickedInfoBox == null)\n\t\t\t\tclickedInfoBox = new InfoBox(clickedInfoBoxOptions);\n\t\t\telse {\n\t\t\t\tclickedInfoBox.setContent(clickedBoxText);\t\t\t\t\t\t\n\t\t\t\tclickedInfoBox.setZIndex(100000);\n\t\t\t}\n\t\t\t\n\t\t\tclickedInfoBox.open(map, marker);\n\t\t}\n\t});\n}\n\nfunction onChangeSortByCategories() {\n\tvar search_text = document.getElementById('search_text').value;\n\tvar search_category = marker_categories.options[marker_categories.selectedIndex].value;\n\t\t\n\tSearchBooks(search_text, search_category);\n}\n\nfunction onSearchBooks(event) {\n\tvar unicode = event.keyCode? event.keyCode : event.charCode;\n\tif (unicode == 13) {\n\t\tvar search_text = document.getElementById('search_text').value;\n\t\tvar search_category = marker_categories.options[marker_categories.selectedIndex].value;\n\t\t\n\t\tSearchBooks(search_text, search_category);\n\t}\n}\n\t</script>\n\t\t<script type=\"text/javascript\" src=\"GoogleMapV3/js/utility.js\"></script>\n\t\t<script type=\"text/javascript\" src=\"GoogleMapV3/js/infobox.js\"></script>\n\t\t\n\t\t<!-- edit by Logan to hopefully make lightbox work for link -->\n\t\t<link rel=\"stylesheet\" href=\"http://thestudentbookproject.org/cache/widgetkit/widgetkit-6232adfb.css\" type=\"text/css\" />\t\n\t\t\n\t\t<!-- edit by Logan to hopefully make lightbox work for link -->\n\n\t\t<script type=\"text/javascript\" src=\"http://thestudentbookproject.org/cache/widgetkit/widgetkit-21519d80.js\"></script>\n\t\t\n\t\t<!--<script src=\"GoogleMapV3/js/data.json\" type=\"text/javascript\"></script>\n\t\t<script type=\"text/javascript\">\n\t\t\tvar script = '<script type=\"text/javascript\" src=\"GoogleMapV3/js/markerclusterer';\n\t\t\tif (document.location.search.indexOf('compiled') !== -1) {\n\t\t\t\tscript += '_compiled';\n\t\t\t}\n\t\t\tscript += '.js\"><' + '/script>';\n\t\t\tdocument.write(script);\n\t\t</script>-->\t\t\n\n\t\t<style type=\"text/css\">\n\t\t\ttable {\n\t\t\t\twidth: 30%;\n\t\t\t}\n\n\t\t\tth {\n\t\t\t\twidth: 30%;\n\t\t\t\ttext-align: left;\n\t\t\t}\n\t\t</style>\n    </head>\n\t\n    <body onload=\"initialize()\" onunload=\"GUnload()\">\n\t\t\n\t\t<div id=\"large_map\" class=\"large_map filters_viewable\">\n\t\t\t<button class=\"filter_rail_toggle\" style=\"width:22px; height:22px; margin-top:0px;\">\n\t\t\t\t<span id=\"controlbtn\" class=\"srp_largemap_imgsheet\" style=\"height:16px;\"></span>\n\t\t\t</button>\n\t\t\n\t\t\t<div id=\"srp_left_rail\" class=\"srp_left_rail less_search_options\">\n\t\t\t\n\t\t\t\t<div id=\"results_listing\">\n\t\t\t\t\n\t\t\t\t\t<div class=\"result_list_actions cf\">\n\t\t\t\t\t\t<div style=\"margin-left:30px; margin-top:0px;\">\n\t\t\t\t\t\t\t<label>Book Search :</label>\n\t\t\t\t\t\t\t<input type=\"text\" id=\"search_text\" name=\"search_text\" onkeyup=\"onSearchBooks(event);\" />\n\t\t\t\t\t\t</div>\n\t\t\t\t\t\t\n\t\t\t\t\t\t<div style=\"margin-left:30px; margin-top:10px; margin-bottom:0px;\">\n\t\t\t\t\t\t\t<label>Categories :</label>\n\t\t\t\t\t\t\t<select id=\"marker_categories\" name=\"marker_categories\" style=\"width:100px; margin-left:10px;\" onchange=\"onChangeSortByCategories();\">\n\t\t\t\t\t\t\t</select>\n\t\t\t\t\t\t</div>\n\t\t\t\t\t\t\n\t\t\t\t\t\t<div style=\"margin-left:30px; margin-top:2px; margin-bottom:0px;\">\n\t\t\t\t\t\t<a data-lightbox=\"width:1000;height:600;\" title=\"Bookstore Price Comparison\" href=\"http://thestudentbookproject.org/Textbook-Price-Comparison/\"><p style=\"font-size:60%;color:gray\">Bookstore Price Comparison</p></a>\n\t\t\t\t\t\t</div>\n\t\t\t\t\t</div>\n\t\t\t\t\t\n\t\t\t\t\t<div id=\"markers_list_section\" style=\"width:270px;\">\n\t\t\t\t\t\t<ul id=\"markers_list\">\n\t\t\t\t\t\t</ul>\n\t\t\t\t\t</div>\n\t\t\t\t\t\n\t\t\t\t\t<div id=\"markers_prev_next_section\" class=\"markers_prev_next\" style=\"white-space: nowrap;\">\n\t\t\t\t\t</div>\n\t\t\t\t\t\n\t\t\t\t</div>\n\t\t\t\t\n\t\t\t</div>\n\t\t\n\t\t\t<div id=\"map_wrapper\" style=\"width:100%; height:800px; position:relative; background: url('GoogleMapV3/images/ajax-loader.gif'); background-repeat:no-repeat;  background-position:center;\">\n\t\t\t\t<div id=\"map_canvas\" style=\"width:100%; height:800px; position:relative; margin-left:300px;\"></div>\n\t\t\t</div>\n\t\t\t\n\t\t</div>\n\t\t\n    </body>\n\t\n</html>\n" ("string")) -> (w20:string)
    n12 = flat-sequence {
      tunnel: w20 -> [w38]
      tunnel: w19 -> [w37]
      tunnel: w7 -> [w36]
      tunnel: w4 -> [w43]
      tunnel: w4 -> [w45]
      tunnel: w7 -> [w44]
      tunnel: [w46] -> w35
      tunnel: [w48] -> w34
      tunnel: [w47] -> w33
      tunnel: w35 -> [w47]
      tunnel: w34 -> [w51]
      tunnel: [w50] -> w32
      tunnel: w33 -> [w50]
      tunnel: w4 -> [w49]
      tunnel: [w53] -> w31
      tunnel: [w52] -> w30
      tunnel: w32 -> [w52]
      tunnel: [w56] -> w29
      tunnel: w31 -> [w56]
      tunnel: [w55] -> w28
      tunnel: w30 -> [w55]
      tunnel: w4 -> [w54]
      tunnel: w29 -> [w58]
      tunnel: w28 -> [w57]
      frame #0 {
        n13 = Write to Text File(file (use dialog)=w37, text=w38) -> ()  [unwired: 2 in, 3 out]
        n14 = call "FTP upload exchange logo.vi"("name of logo"=w36) -> ()  [unwired: 11 in]
      }
      frame #1 {
        n15 = Search and Replace String(replace all?=TRUE ("replace all? (F)"), input string=w43, search string=" ", replace string="_" ("replace string (\"\")")) -> (result string=w39:string)  [unwired: 4 in, 3 out]
        n16 = call "FTP upload HTML map.vi"("Name of Exchange"=w39) -> ()  [unwired: 11 in]
      }
      frame #2 {
        n17 = call "Insert exchange into jos_content.vi"("Image Name"=w44, "title"=w45) -> ()  [unwired: 3 in]
      }
      frame #3 {
        n18 = call "Fetch Last jos_modules ID.vi"() -> ("Last ID"=w46:string)  [unwired: 1 in]
      }
      frame #4 {
        n19 = call "Fetch Last mySQL ID.vi"() -> ("Last ID"=w48:string)  [unwired: 1 in]
      }
      frame #5 {
        n20 = call "Insert book exchange into jos_menu.vi"("id of content article"=w51, "title"=w49) -> ()  [unwired: 3 in]
      }
      frame #6 {
        n21 = call "Fetch Last jos_menu ID.vi"() -> ("Last ID"=w53:string)  [unwired: 1 in]
      }
      frame #7 {
        n22 = call "Insert exchange into jos_modules.vi"("title"=w54) -> ()  [unwired: 4 in]
      }
      frame #8 {
        n23 = call "Insert book exchange into jos_modules_menu.vi"("menuid"=w58, "moduleid"=w57) -> ()  [unwired: 3 in]
      }
    }
  }
